vi "KB-计算数组非零最大值与最小值.vi"(11 "原始数据":dbl[][](array[numeric])) -> (2 "最小值":cluster{"X":dbl, "Y":dbl, "Z":dbl}, 3 "最大值":cluster{"X":dbl, "Y":dbl, "Z":dbl})   [LabVIEW 2015]
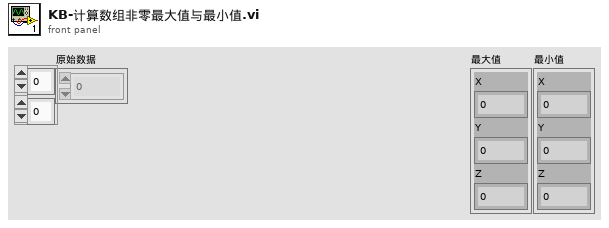
[diagram p1: front panel]
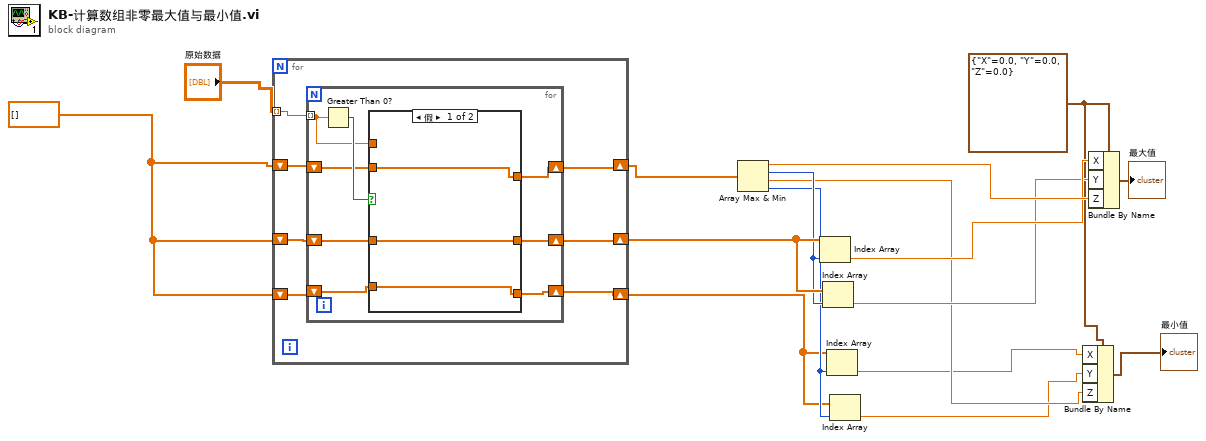
[diagram p0: block diagram]
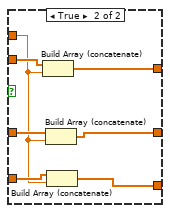
[diagram p2: hidden frame]
diagram:
  w7 = cluster{"X":dbl, "Y":dbl, "Z":dbl} {"X"=0.0, "Y"=0.0, "Z"=0.0}
  w15 = dbl[] []
  n1 = for {
    tunnel: "原始数据" -> [w23] mode=indexing
    shift-right: [w19] -> w14
    shift-left: w15 -> [w22]
    shift-right: [w18] -> w12
    shift-left: w15 -> [w21]
    shift-right: [w17] -> w4
    shift-left: w15 -> [w20]
    n2 = for {
      tunnel: w23 -> [w27] mode=indexing
      shift-right: [w26] -> w19
      shift-left: w22 -> [w30]
      shift-right: [w25] -> w18
      shift-left: w21 -> [w29]
      shift-right: [w24] -> w17
      shift-left: w20 -> [w28]
      n3 = Greater Than 0?(x=w27) -> (x > 0?=w31:bool)
      n4 = case shown="假" w31 {
        tunnel: w30 -> [w34 w41]
        tunnel: w29 -> [w33 w39]
        tunnel: w28 -> [w32 w37]
        tunnel: w27 -> [_ w35]
        tunnel: [w34 w40] -> w26
        tunnel: [w33 w38] -> w25
        tunnel: [w32 w36] -> w24
        frame False {
        }
        frame True {
          n5 = Build Array (concatenate)(w41, w35) -> (w40:dbl[])
          n6 = Build Array (concatenate)(w39, w35) -> (w38:dbl[])
          n7 = Build Array (concatenate)(w37, w35) -> (w36:dbl[])
        }
      }
    }
  }
  n8 = Array Max & Min(array=w14) -> (max value=w13:dbl, max index (indices)=w11:i32, min value=w6:dbl, min index (indices)=w5:i32)
  n9 = Index Array(array=w12, index=w11) -> (element=w10:dbl)
  n10 = Index Array(array=w12, index=w11) -> (element=w9:dbl)
  n11 = Index Array(array=w4, index=w5) -> (element=w2:dbl)
  n12 = Index Array(array=w4, index=w5) -> (element=w1:dbl)
  n13 = Bundle By Name(cluster=w7, "X"=w2, "Y"=w1, "Z"=w6) -> (→"最小值":cluster{"X":dbl, "Y":dbl, "Z":dbl})
  n14 = Bundle By Name(cluster=w7, "X"=w10, "Y"=w9, "Z"=w13) -> (→"最大值":cluster{"X":dbl, "Y":dbl, "Z":dbl})
